vi "W&R(Know Size CRC16 With Data).vi"(0 "VISA resource name in":refnum<visa-resource-name>, 5 "写入指令/数据":string, 7 "总字节数":u32, 9 "超时":u32=1000, 11 "error in":errorcluster) -> (4 "VISA resource name out":refnum<visa-resource-name>, 6 "数据":string, 15 "error out":errorcluster)   [LabVIEW 2018]
uses:
  <vilib>/Instr/_visa.llb/VISA Set IO Buffer Mask.ctl
  <vilib>/Instr/_visa.llb/VISA Flush IO Buffer Mask.ctl
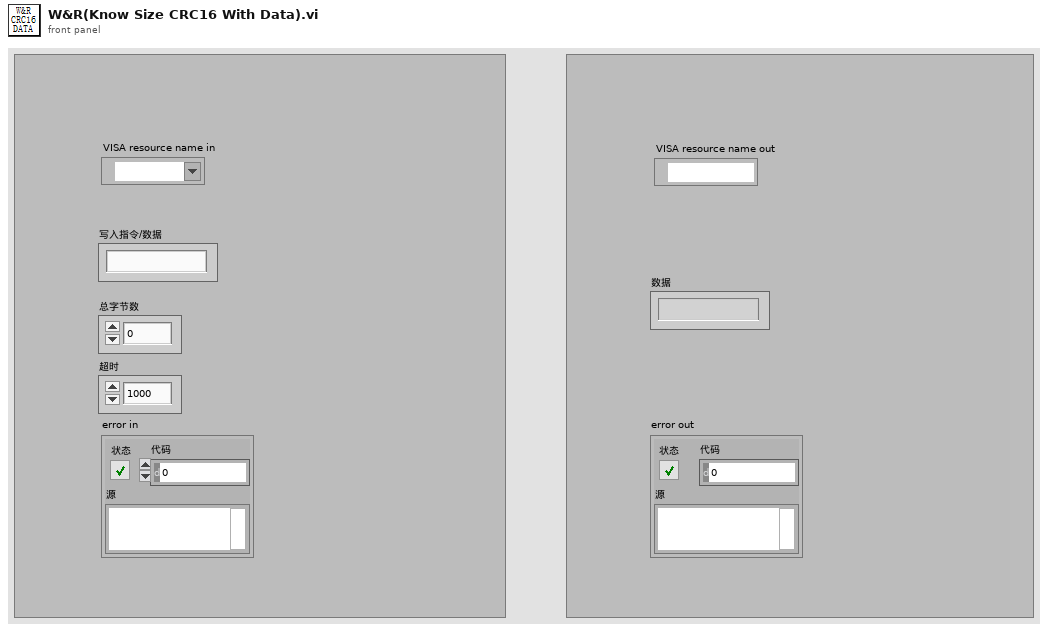
[diagram p1: front panel]
types:
  T1 = typedef "VISA Flush IO Buffer Mask.ctl" = u16
  T2 = typedef "VISA Set IO Buffer Mask.ctl" = u16
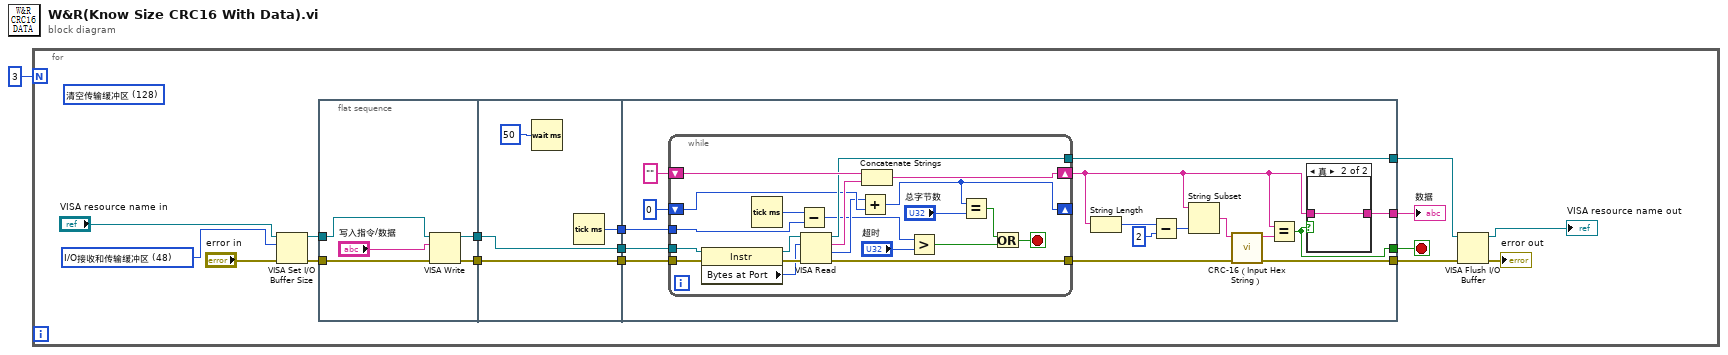
[diagram p0: block diagram]
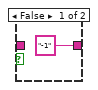
[diagram p2: hidden frame]
diagram:
  n1 = for {
    N: 3 -> [_]
    stop <- w13 stop-if-true
    (unwired) T1 128 items=["清空接收缓冲区"=16, "向设备写入传输缓冲区"=32, "清空接收缓冲区（无I/O）"=64, "清空传输缓冲区"=128] ("Mask")
    w10 = T2 48 items=["I/O接收缓冲区"=16, "I/O传输缓冲区"=32, "I/O接收和传输缓冲区"=48] ("Mask")
    n2 = VISA Set I/O Buffer Size(VISA resource name="VISA resource name in", mask (16)=w10, error in (no error)="error in") -> (VISA resource name out=w8:refnum<visa-resource-name>, error out=w6:errorcluster)  [unwired: 1 in]
    n3 = flat-sequence {
      tunnel: w8 -> [w22]
      tunnel: [w21] -> w17
      tunnel: [w19] -> w16
      tunnel: w6 -> [w18]
      tunnel: [w26] -> w15
      tunnel: w17 -> [w26]
      tunnel: [w25] -> w14
      tunnel: w16 -> [w25]
      tunnel: [w24] -> w12
      tunnel: w15 -> [w42]
      tunnel: w14 -> [w41]
      tunnel: [w29] -> w13
      tunnel: [w40] -> w5
      tunnel: [w30] -> w4
      tunnel: w12 -> [w37]
      tunnel: [w27] -> w11
      frame #0 {
        n4 = VISA Write(VISA resource name=w22, write buffer="写入指令/数据", error in (no error)=w18) -> (VISA resource name out=w21:refnum<visa-resource-name>, error out=w19:errorcluster)  [unwired: 1 out]
      }
      frame #1 {
        n5 = Wait (ms)(milliseconds to wait=u32 50 ("等待时间（毫秒）")) -> ()  [unwired: 1 out]
        n6 = Tick Count (ms)() -> (millisecond timer value=w24:u32)
      }
      frame #2 {
        n7 = while {
          tunnel: w42 -> [w65]
          tunnel: w41 -> [w64]
          shift-right: [w61] -> w28
          shift-left: "" -> [w60]
          tunnel: [w59] -> w40
          tunnel: [w58] -> w31
          shift-right: [w54] -> _
          shift-left: u32 0 -> [w55]
          tunnel: w37 -> [w51]
          stop <- w47 stop-if-true
          n8 = property class="Instr"(reference=w65, error in=w64) -> (reference out=w63:refnum<visa-resource-name>, error out=w62:errorcluster, "Bytes at Port"=w56:u32)
          n9 = Tick Count (ms)() -> (millisecond timer value=w52:u32)
          n10 = Subtract(x=w52, y=w51) -> (x-y=w50:u32)
          n11 = VISA Read(VISA resource name=w63, byte count=w56, error in (no error)=w62) -> (VISA resource name out=w59:refnum<visa-resource-name>, read buffer=w57:string, return count=w53:u32, error out=w58:errorcluster)
          n12 = Add(x=w53, y=w55) -> (x+y=w54:u32)
          n13 = Concatenate Strings(w60, w57) -> (w61:string)
          n14 = Greater?(x=w50, y="超时") -> (0:w48:bool)
          n15 = Equal?(x=w54, y="总字节数") -> (x = y?=w49:bool)
          n16 = Or(x=w49, y=w48) -> (x .or. y?=w47:bool)
        }
        n17 = String Length(string=w28) -> (length=w36:i32)
        n18 = Subtract(x=w36, y=2) -> (x-y=w34:i32)
        n19 = String Subset(string=w28, length (rest)=w34) -> (substring=w33:string)  [unwired: 1 in]
        n20 = call "CRC-16（Input Hex String）.vi"("error in (no error)"=w31, "发送数据"=w33) -> ("error out"=w30:errorcluster, "完整命令"=w32:string)  [unwired: 8 in]
        n21 = Equal?(x=w28, y=w32) -> (x = y?=w29:bool)
        n22 = case shown="真" w29 {
          tunnel: w28 -> [_ w44]
          tunnel: ["-1" w44] -> w27
          frame False {
          }
          frame True {
          }
        }
      }
    }
    n23 = VISA Flush I/O Buffer(VISA resource name=w5, error in (no error)=w4) -> (VISA resource name out=→"VISA resource name out":refnum<visa-resource-name>, error out=→"error out":errorcluster)  [unwired: 1 in]
    "数据" <- w11
  }
